vi "proj_wstaw_1.vi"(9 "Kolumna":i32, 10 "Wiersz":i32, 11 "Plansza":i32[][](array[numeric])) -> (3 "Plansza sprawdzajaca":i32[][](array[numeric]))   [LabVIEW 2020]
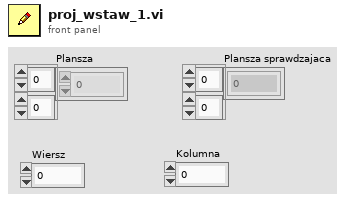
[diagram p1: front panel]
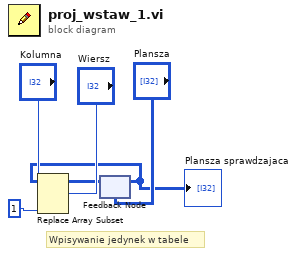
[diagram p0: block diagram]
diagram:
  # "Wpisywanie jedynek w tabele"
  n1 = feedback #1("Plansza") -> (w3:i32[][])
  "Plansza sprawdzajaca" <- w3
  n2 = Replace Array Subset(array=w3, new element=1 ("new element/subarray"), index (row)="Wiersz", index (col)="Kolumna") -> (w2:i32[][])
  n3 = feedback-in #1(w2) -> ()
